vi "CANOpen Import PDO.vi"(8 "error in (no error)":errorcluster, 11 "PDO in":T1[](array[typedef]) {"Bit Offset" max=8 step=1; "Byte Offset" max=8 step=1}) -> (0 "error out":errorcluster, 3 "PDO out":T1[](array[typedef]) {"Bit Offset" max=8 step=1; "Byte Offset" max=8 step=1})   [LabVIEW 2021, in "CANOpen Addon System Explorer.lvlib"]
uses:
  CANOpen Addon System Explorer.lvlib
  Shared/CANOpen_PDO Parameter Settings.ctl
  Shared/CANOpen_PDO Data Type.ctl
  CANopen Byte Order.ctl
  Shared/CANOpen Addon Shared.lvlib
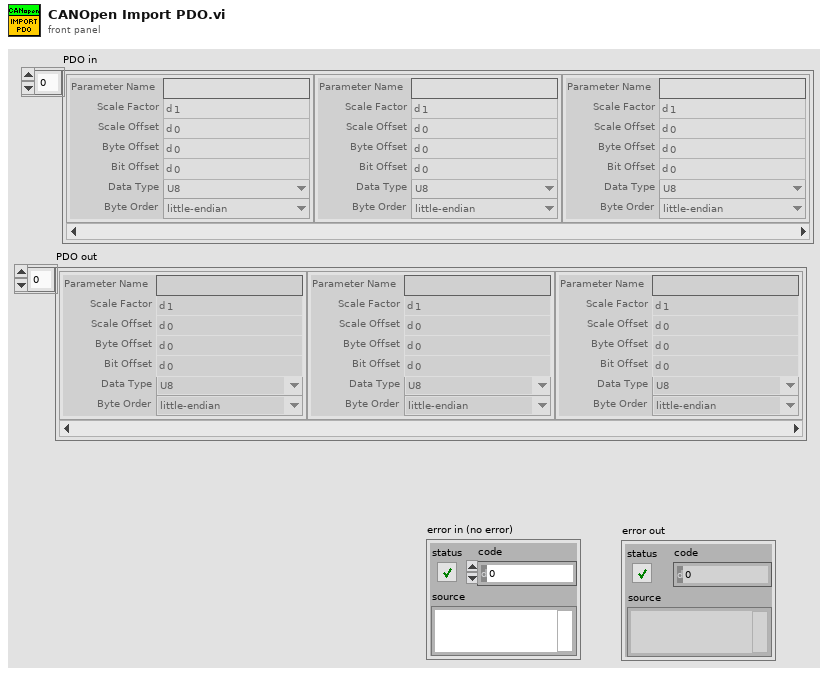
[diagram p1: front panel]
types:
  T1 = typedef "CANOpen Addon Shared.lvlib/CANOpen_PDO Parameter Settings.ctl" = cluster{"Parameter Name":string, "Scale Factor":dbl, "Scale Offset":dbl, "Byte Offset":u8, "Bit Offset":u8, "Data Type":T2, "Byte Order":T3}
  T2 = typedef "CANOpen Addon Shared.lvlib/CANOpen_PDO Data Type.ctl" = enum16{"U8", "U16", "U32", "I8", "I16", "I32", "Single", "Double", "Boolean"}
  T3 = typedef "CANOpen Addon System Explorer.lvlib/CANopen Byte Order.ctl" = enum16{"big-endian network order", "little-endian"}
  T4 = enum16{"big-endian network order", "little-endian"}
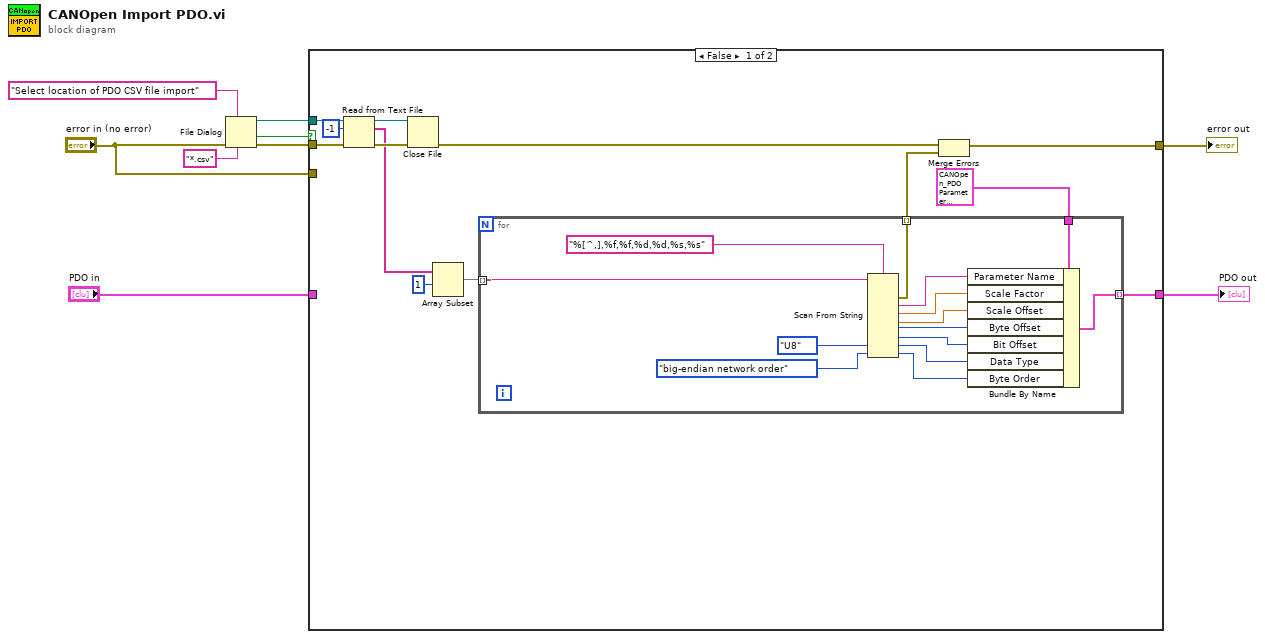
[diagram p0: block diagram]
diagram:
  n1 = File Dialog(6:"*.csv" ("pattern (all files)"), 7:"Select location of PDO CSV file import" ("prompt"), 8:"error in (no error)") -> (0:w6:errorcluster, 1:w7:bool, 3:w3:path)  [unwired: 4 in, 1 out]
  n2 = case shown="False" w7 {
    tunnel: w6 -> [w21 _]
    tunnel: [w12 w38] -> w5
    tunnel: "error in (no error)" -> [_ w38]
    tunnel: w3 -> [w22 _]
    tunnel: "PDO in" -> [_ w37]
    tunnel: [w19 w37] -> w1
    frame False {
      n3 = Read from Text File(file (use dialog)=w22, count=-1, error in=w21) -> (refnum out=w15:refnum<file>, text=w14:string[], error out=w16:errorcluster)  [unwired: 2 out]
      n4 = Close File(refnum=w15, error in=w16) -> (error out=w20:errorcluster)  [unwired: 1 out]
      n5 = Array Subset(array=w14, index=1) -> (w10:string[])  [unwired: 1 in]
      n6 = for {
        tunnel: T1 {"Parameter Name"="", "Scale Factor"=1.0, "Scale Offset"=0.0, "Byte Offset"=0, "Bit Offset"=0, "Data Type"=enum."U8", "Byte Order"=enum."little-endian"} ("System Cluster") -> [w36]
        tunnel: w10 -> [w25] mode=indexing
        tunnel: [w27] -> w19 mode=indexing
        tunnel: [w26] -> w11 mode=indexing
        n7 = Scan From String(format string="%[^,],%f,%f,%d,%d,%s,%s", input string=w25, default 6=CANOpen_PDO_Data_Type."U8" ("Data Type"), default 7=T4."big-endian network order" ("Byte Order")) -> (error out=w26:errorcluster, output 1=w23:string, output 2=w35:dbl, output 3=w34:dbl, output 4=w33:i32, output 5=w32:i32, output 6=w30:T2, output 7=w28:T4)  [unwired: 7 in, 2 out]
        n8 = Bundle By Name(cluster=w36, "Parameter Name"=w23, "Scale Factor"=w35, "Scale Offset"=w34, "Byte Offset"=w33, "Bit Offset"=w32, "Data Type"=w30, "Byte Order"=w28) -> (w27:T1)
      }
      n9 = Merge Errors(w20, w11) -> (w12:errorcluster)
    }
    frame True {
    }
  }
  "PDO out" <- w1
  "error out" <- w5
